vi "DVRAccess.vi"() -> ()   [LabVIEW 2023]
doc: "This Vi demonstrates the behaviour of DVR."
panel:
  in  "error in (no error)":errorcluster
  out "error out":errorcluster
  in  "stop":bool
  out "Data value":dbl
  # "Instructions:\n\n-> Run the Vi and observe the behaviour of DVR.\n-> Make changes in delay times in block diagram and\n      observe the behaviour.\n-> Press STOP to stop the running vi."
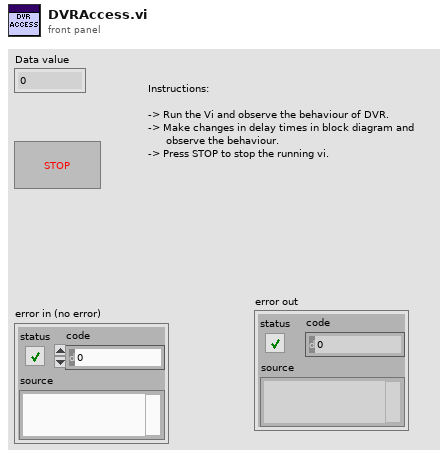
[diagram p1: front panel]
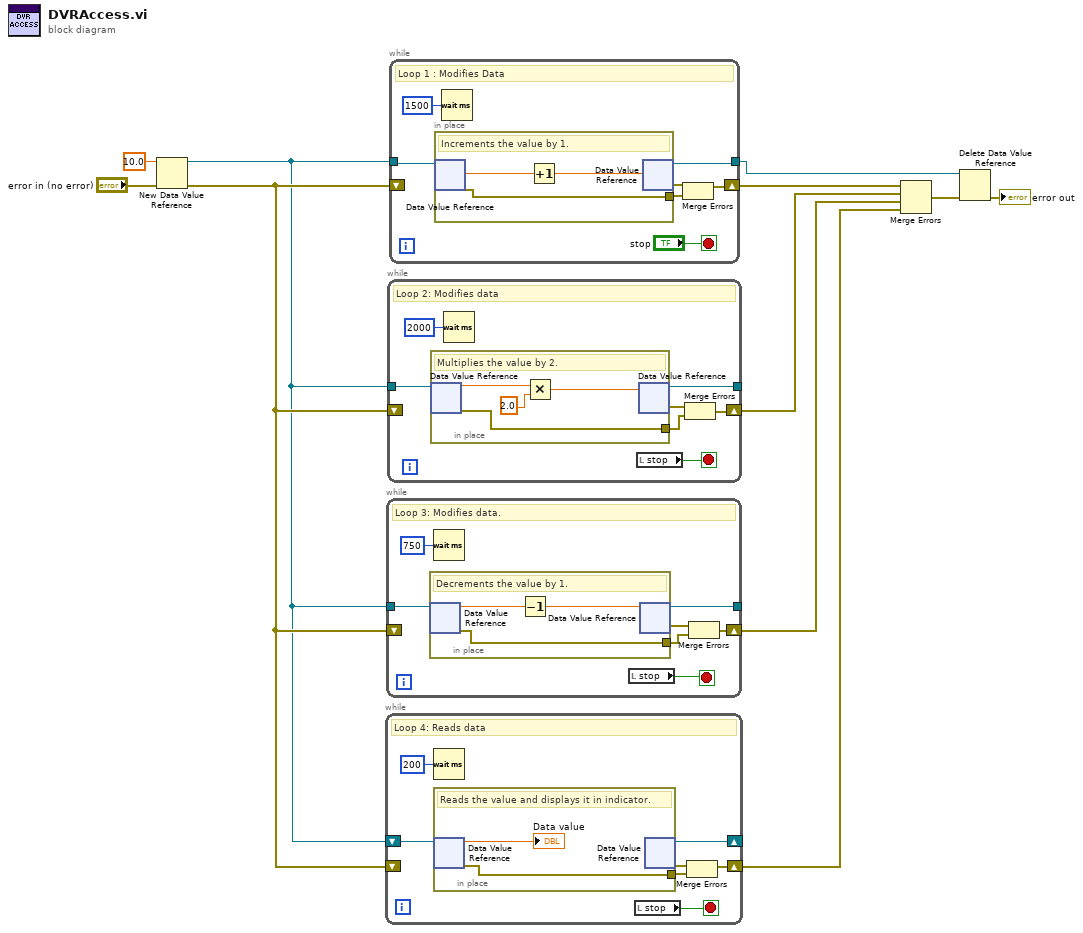
[diagram p0: block diagram]
diagram:
  n1 = New Data Value Reference(data value=10.0, error in="error in (no error)") -> (data value reference=w2:refnum<data-value>, error out=w10:errorcluster)
  n2 = while {
    shift-right: [w13] -> w6
    shift-left: w10 -> [_]
    shift-right: [w15] -> _
    shift-left: w2 -> [w18]
    stop <- w17 stop-if-true
    # "Loop 4: Reads data"
    n3 = Wait (ms)(milliseconds to wait=u32 200) -> ()  [unwired: 1 out]
    n4 = in-place {
      in-place-border: [w19] -> w12
      # "Reads the value and displays it in indicator."
      n5 = in-place-dvr #1(w18) -> (→"Data value":dbl, w19:errorcluster)
      n6 = in-place-dvr #1() -> (w15:refnum<data-value>, w14:errorcluster)  [unwired: 1 in]
    }
    n7 = local read "stop"() -> (w17:bool)
    n8 = Merge Errors(w14, w12) -> (w13:errorcluster)
  }
  n9 = while {
    shift-right: [w23] -> w7
    shift-left: w10 -> [_]
    tunnel: w2 -> [w27]
    tunnel: [w24] -> _
    stop <- w26 stop-if-true
    # "Loop 3: Modifies data."
    n10 = in-place {
      in-place-border: [w28] -> w21
      # "Decrements the value by 1."
      n11 = in-place-dvr #2(w27) -> (w30:dbl, w28:errorcluster)
      n12 = Decrement(x=w30) -> (x-1=w29:dbl)
      n13 = in-place-dvr #2(w29) -> (w24:refnum<data-value>, w22:errorcluster)
    }
    n14 = Wait (ms)(milliseconds to wait=u32 750) -> ()  [unwired: 1 out]
    n15 = local read "stop"() -> (w26:bool)
    n16 = Merge Errors(w22, w21) -> (w23:errorcluster)
  }
  n17 = while {
    shift-right: [w33] -> w8
    shift-left: w10 -> [_]
    tunnel: w2 -> [w37]
    tunnel: [w34] -> _
    stop <- w36 stop-if-true
    # "Loop 2: Modifies data"
    n18 = in-place {
      in-place-border: [w38] -> w31
      # "Multiplies the value by 2."
      n19 = in-place-dvr #3(w37) -> (w41:dbl, w38:errorcluster)
      n20 = Multiply(x=w41, y=2.0) -> (x*y=w39:dbl)
      n21 = in-place-dvr #3(w39) -> (w34:refnum<data-value>, w32:errorcluster)
    }
    n22 = Wait (ms)(milliseconds to wait=u32 2000) -> ()  [unwired: 1 out]
    n23 = local read "stop"() -> (w36:bool)
    n24 = Merge Errors(w32, w31) -> (w33:errorcluster)
  }
  n25 = while {
    shift-right: [w43] -> w9
    shift-left: w10 -> [_]
    tunnel: w2 -> [w45]
    tunnel: [w46] -> w3
    stop <- "stop" stop-if-true
    # "Loop 1 : Modifies Data"
    n26 = in-place {
      in-place-border: [w49] -> w42
      # "Increments the value by 1."
      n27 = in-place-dvr #4(w45) -> (w51:dbl, w49:errorcluster)
      n28 = Increment(x=w51) -> (x+1=w50:dbl)
      n29 = in-place-dvr #4(w50) -> (w46:refnum<data-value>, w44:errorcluster)
    }
    n30 = Wait (ms)(milliseconds to wait=u32 1500) -> ()  [unwired: 1 out]
    n31 = Merge Errors(w44, w42) -> (w43:errorcluster)
  }
  n32 = Merge Errors(w9, w8, w7, w6) -> (w5:errorcluster)
  n33 = Delete Data Value Reference(data value reference=w3, error in=w5) -> (error out=→"error out":errorcluster)  [unwired: 1 out]
